vi "niFpgaScaledWinInsideSCTLIndex.vi"(0 "real data in":fxp<+/-,24,1>, 5 "imaginary data in":fxp<+/-,24,1>, 7 "coefficient index":u16, 9 "input valid":bool, 12 "ready for output":bool) -> (3 "data index":u16, 4 "real data out":fxp<+/-,24,-1>, 6 "imaginary data out":fxp<+/-,24,-1>, 10 "output valid":bool, 14 "ready for input":bool)   [LabVIEW 2017]
uses:
  <vilib>/rvi/FXPMathLib/basic elements/FxpDiscreteDelay/XNode/nifxpmath_DiscreteDelay.xnode
  <vilib>/rvi/FXPMathLib/FxpMul/XNode/nifxpmath_Multiplier.xnode
  <vilib>/rvi/FXPMathLib/sim/FxpSim.dll
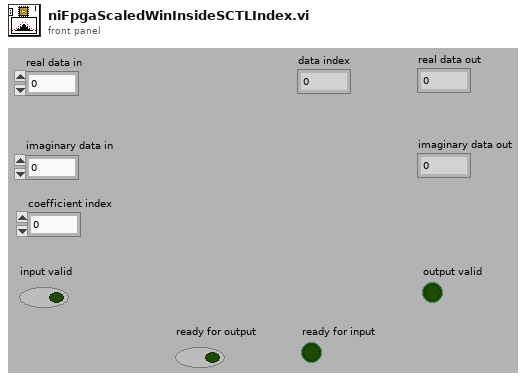
[diagram p1: front panel]
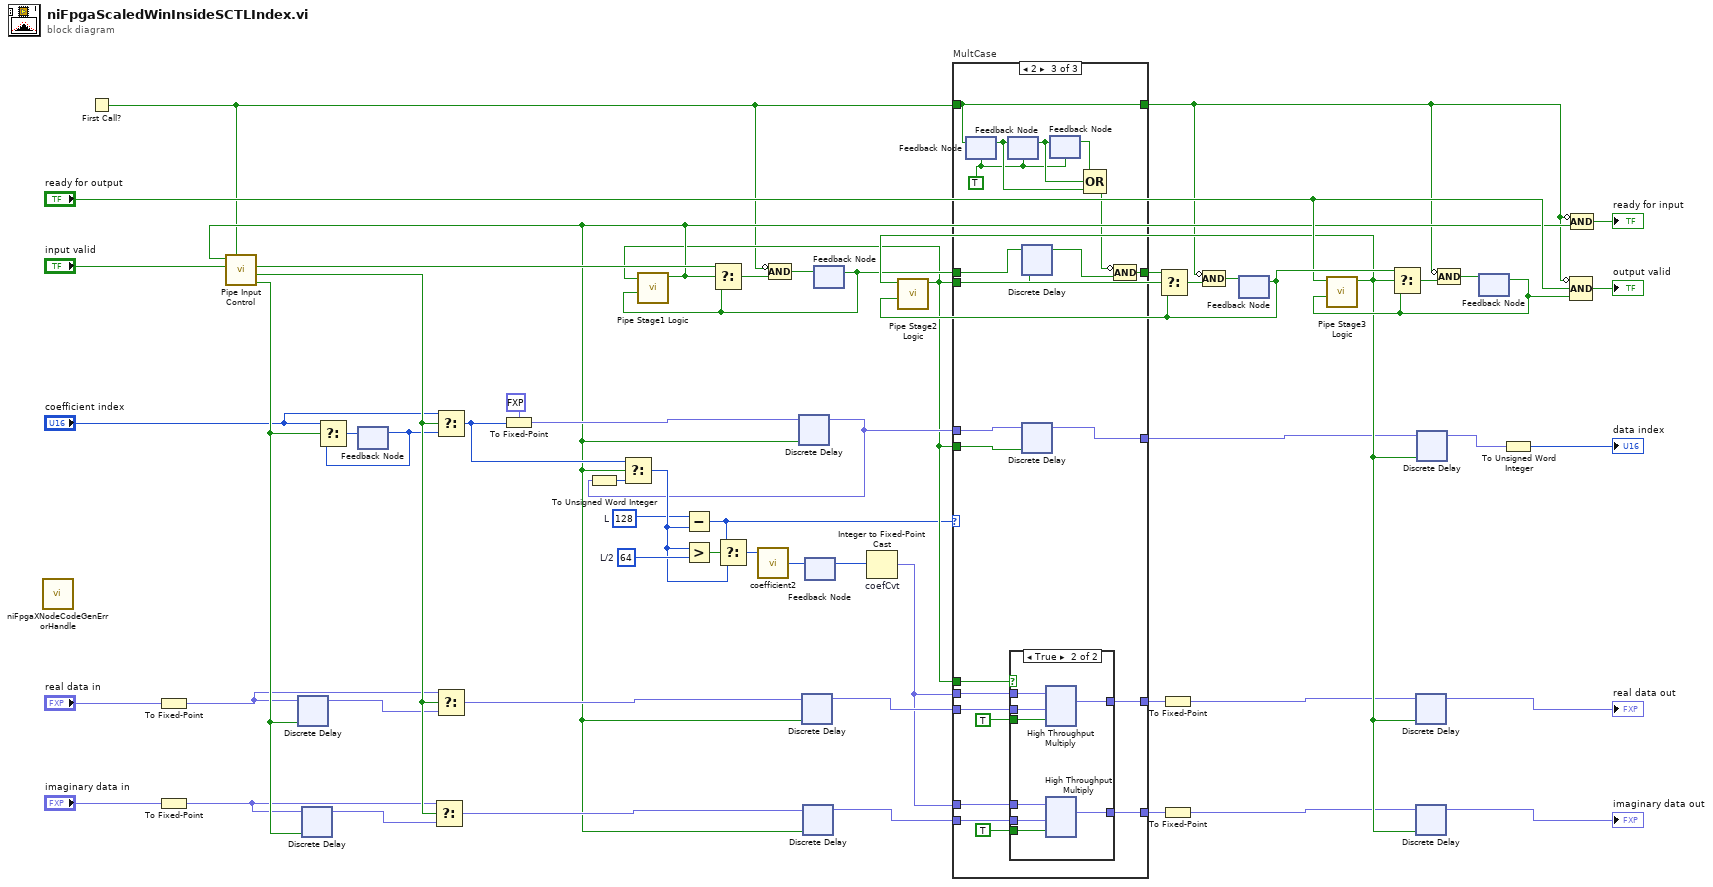
[diagram p0: block diagram]
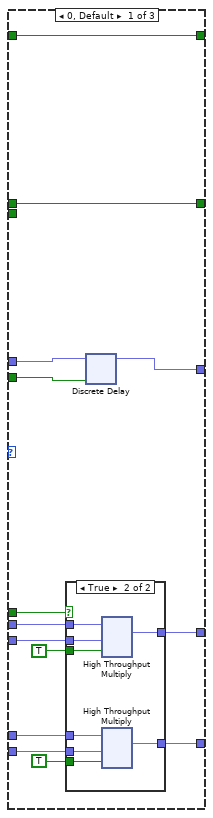
[diagram p2: hidden frame]
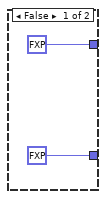
[diagram p3: hidden frame]
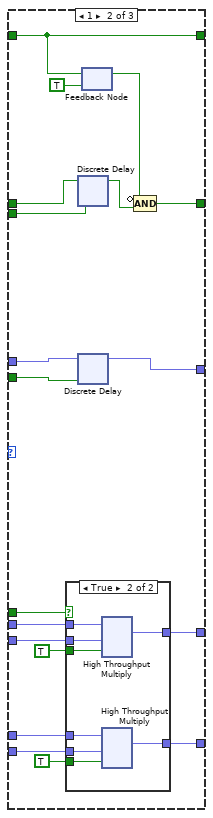
[diagram p4: hidden frame]
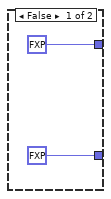
[diagram p5: hidden frame]
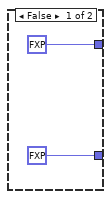
[diagram p6: hidden frame]
diagram:
  w41 = u16 128  # L
  w46 = u16 64  # L/2
  n1 = call <vilib>:"niFpgaXNodeCodeGenErrorHandle.vi"() -> ()  [unwired: 1 in]
  n2 = First Call?() -> (First Call?: T/F=w17:bool)
  n3 = To Fixed-Point(number="real data in") -> (fixed-point=w3:fxp<+/-,24,1>)  [unwired: 1 in]
  n4 = To Fixed-Point(number="imaginary data in") -> (fixed-point=w5:fxp<+/-,24,1>)  [unwired: 1 in]
  n5 = feedback #1() -> (w11:u16)  [unwired: 1 out]
  n6 = feedback #2() -> (w2:i32)  [unwired: 1 out]
  n7 = feedback #3() -> (w20:bool)  [unwired: 1 out]
  n8 = Integer to Fixed-Point Cast "coefCvt"(integer=w2) -> (fixed-point=w1:fxp<+/-,32,32>)  [unwired: 1 in]
  n9 = feedback #4() -> (w51:bool)  [unwired: 1 out]
  n10 = feedback #5() -> (w50:bool)  [unwired: 1 out]
  n11 = call "Pipe Stage3 Logic"("last output valid"=w50, "ready for output"="ready for output") -> ("ready For input"=w27:bool)  [unwired: 9 out]
  n12 = call "Pipe Stage2 Logic"("last output valid"=w51, "ready for output"=w27) -> ("ready For input"=w18:bool)  [unwired: 9 out]
  n13 = call "Pipe Stage1 Logic"("last output valid"=w20, "ready for output"=w18) -> ("ready For input"=w25:bool)  [unwired: 9 out]
  n14 = call "Pipe Input Control"("reset"=w17, "input valid"="input valid", "ready for input"=w25) -> ("input buffer enable"=w34:bool, "Input Mux Sel"=w37:bool, "output valid"=w58:bool)  [unwired: 6 out]
  n15 = xnode "Discrete Delay"("D"=w3, "enable"=w34) -> ("Q"=w35:fxp<+/-,24,1>)
  n16 = xnode "Discrete Delay"("D"=w5, "enable"=w34) -> ("Q"=w33:fxp<+/-,24,1>)
  n17 = Select(t="coefficient index", s=w34, f=w11) -> (s? t:f=w10:u16)
  n18 = feedback-in #1(w10) -> ()
  n19 = Select(t=w5, s=w37, f=w33) -> (s? t:f=w31:fxp<+/-,24,1>)
  n20 = Select(t="coefficient index", s=w37, f=w11) -> (s? t:f=w40:u16)
  n21 = Select(t=w3, s=w37, f=w35) -> (s? t:f=w32:fxp<+/-,24,1>)
  n22 = To Fixed-Point(fixed-point type=fxp<+,7,7> 0.0 ("LBitMask"), number=w40) -> (fixed-point=w26:fxp<+,7,7>)
  n23 = Select(t=w58, s=w25, f=w20) -> (s? t:f=w57:bool)
  n24 = Compound Arithmetic op=AND(invert w17, w57) -> (w56:bool)
  n25 = xnode "Discrete Delay"("D"=w26, "enable"=w25) -> ("Q"=w24:fxp<+,7,7>)
  n26 = To Unsigned Word Integer(number=w24) -> (unsigned 16bit integer=w42:u16)
  n27 = Select(t=w40, s=w25, f=w42) -> (s? t:f=w44:u16)
  n28 = Subtract(x=w41, y=w44) -> (x-y=w7:u16)
  n29 = Greater?(x=w44, y=w46) -> (0:w47:bool)
  n30 = Select(t=w7, s=w47, f=w44) -> (s? t:f=w43:u16)
  n31 = call "coefficient2"("address"=w43) -> ("data out"=w45:i32)  [unwired: 8 in]
  n32 = xnode "Discrete Delay"("D"=w32, "enable"=w25) -> ("Q"=w22:fxp<+/-,24,1>)
  n33 = xnode "Discrete Delay"("D"=w31, "enable"=w25) -> ("Q"=w21:fxp<+/-,24,1>)
  n34 = feedback-in #2(w45) -> ()
  n35 = feedback-in #3(w56) -> ()
  n36 = case "MultCase" shown="2" w7 {
    tunnel: w24 -> [w72 w101 w133]
    tunnel: w18 -> [w71 w100 w132]
    tunnel: [w70 w99 w131] -> w23
    tunnel: w1 -> [w69 w98 w130]
    tunnel: w22 -> [w68 w97 w129]
    tunnel: w1 -> [w67 w96 w128]
    tunnel: w21 -> [w66 w95 w127]
    tunnel: [w60 w84 w114] -> w15
    tunnel: [w61 w85 w115] -> w13
    tunnel: w18 -> [w65 w94 w126]
    tunnel: w20 -> [w64 w92 w125]
    tunnel: [w64 w89 w123] -> w19
    tunnel: w18 -> [_ w88 w122]
    tunnel: w17 -> [w59 w83 w113]
    tunnel: [w59 w83 w113] -> w16
    frame 0, Default {
      n37 = case shown="True" w65 {
        tunnel: w69 -> [_ w82]
        tunnel: w68 -> [_ w81]
        tunnel: [fxp<+,1,1> 0.0 w80] -> w61
        tunnel: w67 -> [_ w79]
        tunnel: w66 -> [_ w78]
        tunnel: [fxp<+,1,1> 0.0 w77] -> w60
        tunnel: TRUE -> [_ w76]
        tunnel: TRUE -> [_ w75]
        frame False {
        }
        frame True {
          n38 = xnode "High Throughput Multiply"("x"=w82, "y"=w81, "input valid"=w76) -> ("x*y"=w80:fxp<+/-,56,33>)  [unwired: 1 in, 2 out]
          n39 = xnode "High Throughput Multiply"("x"=w79, "y"=w78, "input valid"=w75) -> ("x*y"=w77:fxp<+/-,56,33>)  [unwired: 1 in, 2 out]
        }
      }
      n40 = xnode "Discrete Delay"("D"=w72, "enable"=w71) -> ("Q"=w70:fxp<+,7,7>)
    }
    frame 1 {
      n41 = case shown="True" w94 {
        tunnel: w98 -> [_ w111]
        tunnel: w97 -> [_ w110]
        tunnel: [fxp<+,1,1> 0.0 w109] -> w85
        tunnel: w96 -> [_ w108]
        tunnel: w95 -> [_ w107]
        tunnel: [fxp<+,1,1> 0.0 w106] -> w84
        tunnel: TRUE -> [_ w105]
        tunnel: TRUE -> [_ w104]
        frame False {
        }
        frame True {
          n42 = xnode "High Throughput Multiply"("x"=w111, "y"=w110, "input valid"=w105) -> ("x*y"=w109:fxp<+/-,56,33>)  [unwired: 1 in, 2 out]
          n43 = xnode "High Throughput Multiply"("x"=w108, "y"=w107, "input valid"=w104) -> ("x*y"=w106:fxp<+/-,56,33>)  [unwired: 1 in, 2 out]
        }
      }
      n44 = xnode "Discrete Delay"("D"=w92, "enable"=w88) -> ("Q"=w91:bool)
      n45 = xnode "Discrete Delay"("D"=w101, "enable"=w100) -> ("Q"=w99:fxp<+,7,7>)
      n46 = feedback-in #6(w83) -> ()
      n47 = feedback #6(TRUE ("First Call?: T/F")) -> (w90:bool)
      n48 = Compound Arithmetic op=AND(invert w90, w91) -> (w89:bool)
    }
    frame 2 {
      w112 = TRUE ("First Call?: T/F")
      n49 = feedback-in #7(w113) -> ()
      n50 = feedback #7(w112) -> (w119:bool)
      n51 = feedback-in #8(w119) -> ()
      n52 = feedback #8(w112) -> (w120:bool)
      n53 = case shown="True" w126 {
        tunnel: w130 -> [_ w143]
        tunnel: w129 -> [_ w142]
        tunnel: [fxp<+,1,1> 0.0 w141] -> w115
        tunnel: w128 -> [_ w140]
        tunnel: w127 -> [_ w139]
        tunnel: [fxp<+,1,1> 0.0 w138] -> w114
        tunnel: TRUE -> [_ w137]
        tunnel: TRUE -> [_ w136]
        frame False {
        }
        frame True {
          n54 = xnode "High Throughput Multiply"("x"=w143, "y"=w142, "input valid"=w137) -> ("x*y"=w141:fxp<+/-,56,33>)  [unwired: 1 in, 2 out]
          n55 = xnode "High Throughput Multiply"("x"=w140, "y"=w139, "input valid"=w136) -> ("x*y"=w138:fxp<+/-,56,33>)  [unwired: 1 in, 2 out]
        }
      }
      n56 = xnode "Discrete Delay"("D"=w125, "enable"=w122) -> ("Q"=w124:bool)
      n57 = xnode "Discrete Delay"("D"=w133, "enable"=w132) -> ("Q"=w131:fxp<+,7,7>)
      n58 = feedback-in #9(w120) -> ()
      n59 = feedback #9(w112) -> (w121:bool)
      n60 = Compound Arithmetic op=OR(w121, w120, w119) -> (w118:bool)
      n61 = Compound Arithmetic op=AND(invert w118, w124) -> (w123:bool)
    }
  }
  n62 = Select(t=w19, s=w18, f=w51) -> (s? t:f=w55:bool)
  n63 = To Fixed-Point ("MultCast")(number=w13) -> (fixed-point=w12:fxp<+/-,24,-1>)  [unwired: 1 out]
  n64 = To Fixed-Point ("MultCast")(number=w15) -> (fixed-point=w14:fxp<+/-,24,-1>)  [unwired: 1 out]
  n65 = Compound Arithmetic op=AND(invert w16, w55) -> (w54:bool)
  n66 = feedback-in #4(w54) -> ()
  n67 = Select(t=w51, s=w27, f=w50) -> (s? t:f=w52:bool)
  n68 = xnode "Discrete Delay"("D"=w12, "enable"=w27) -> ("Q"=→"real data out":fxp<+/-,24,-1>)
  n69 = xnode "Discrete Delay"("D"=w14, "enable"=w27) -> ("Q"=→"imaginary data out":fxp<+/-,24,-1>)
  n70 = xnode "Discrete Delay"("D"=w23, "enable"=w27) -> ("Q"=w28:fxp<+,7,7>)
  n71 = Compound Arithmetic op=AND(invert w16, w52) -> (w53:bool)
  n72 = feedback-in #5(w53) -> ()
  n73 = To Unsigned Word Integer(number=w28) -> (unsigned 16bit integer=→"data index":u16)
  n74 = Compound Arithmetic op=AND(invert w16, "ready for output", w50) -> (→"output valid":bool)
  n75 = Compound Arithmetic op=AND(invert w16, w25) -> (→"ready for input":bool)
